vi "IT6900 Run List.vi"() -> ()   [LabVIEW 2013]
uses:
  IT6900.lvlib
panel:
  in  "List Step Count":i32=2 min=1
  in  "Loop count":i32=1 min=0
  in  "List Timer":i32=3 min=0
  in  "Trigger Current Limit (0.0 A)":dbl format="%.2g"
  in  "Trigger Voltage Limit (0.0 V)":dbl format="%.2g"
  in  "List Save Region":i8 min=0 max=9
  in  "Serial Configuration":T1={"Baud Rate"=9600, "Parity"=0, "Data Bits"=8, "Stop Bits"=10, "Flow Control"=0} {"Flow Control" items=["None", "XON/XOFF", "RTS/CTS", "XON/XOFF & RTS/CTS", "DTR/DSR", "XON/XOFF & DTR/DSR"]; "Stop Bits" items=["1.0"=10, "1.5"=15, "2.0"=20]; "Data Bits" items=["7"=7, "8"=8]; "Parity" items=["None", "Odd", "Even", "Mark", "Space"]; "Baud Rate" items=["300"=300, "600"=600, "1200"=1200, "2400"=2400, "4800"=4800, "9600"=9600, "19200"=19200]}
  in  "VISA resource name":refnum<visa-resource-name>
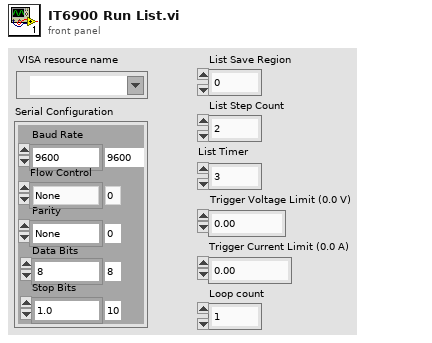
[diagram p1: front panel]
types:
  T1 = cluster{"Baud Rate":u32, "Parity":u16, "Data Bits":u16, "Stop Bits":u16, "Flow Control":u16}
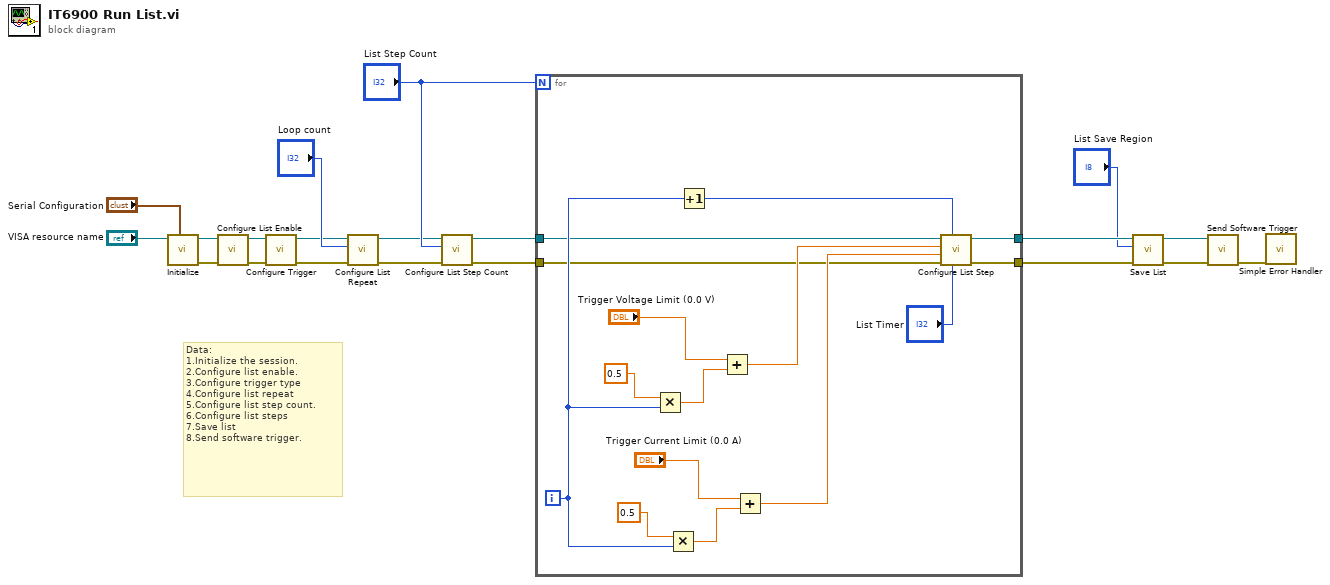
[diagram p0: block diagram]
diagram:
  # "Data:\n1.Initialize the session.\n2.Configure list enable.\n3.Configure trigger type\n4.Configure list repeat\n5.Configure list step count.\n6.Configure list steps\n7.Save list\n8.Send software trigger."
  n1 = call "Initialize.vi"("Serial Configuration"="Serial Configuration", "VISA resource name"="VISA resource name") -> ("error out"=w9:errorcluster, "VISA resource name out"=w10:refnum<visa-resource-name>)  [unwired: 8 in]
  n2 = call "Configure List Enable.vi"("error in (no error)"=w9, "VISA resource name"=w10) -> ("error out"=w8:errorcluster, "VISA resource name out"=w7:refnum<visa-resource-name>)  [unwired: 8 in]
  n3 = call "Configure Trigger.vi"("error in (no error)"=w8, "VISA resource name"=w7) -> ("error out"=w5:errorcluster, "VISA resource name out"=w6:refnum<visa-resource-name>)  [unwired: 8 in]
  n4 = call "Configure List Repeat.vi"("error in (no error)"=w5, "Loop count (1)"="Loop count", "VISA resource name"=w6) -> ("error out"=w3:errorcluster, "VISA resource name out"=w4:refnum<visa-resource-name>)  [unwired: 7 in]
  n5 = call "Configure List Step Count.vi"("error in (no error)"=w3, "List Total"="List Step Count", "VISA resource name"=w4) -> ("error out"=w12:errorcluster, "VISA resource name out"=w13:refnum<visa-resource-name>)  [unwired: 7 in]
  n6 = for {
    N: "List Step Count" -> [_]
    tunnel: w13 -> [w25]
    tunnel: w12 -> [w24]
    tunnel: [w23] -> w18
    tunnel: [w22] -> w17
    i -> [w27]
    n7 = Multiply(x=0.5, y=w27) -> (x*y=w34:dbl)
    n8 = Multiply(x=0.5, y=w27) -> (x*y=w30:dbl)
    n9 = Increment(x=w27) -> (x+1=w26:i32)
    n10 = Add(x="Trigger Voltage Limit (0.0 V)", y=w34) -> (x+y=w32:dbl)
    n11 = Add(x="Trigger Current Limit (0.0 A)", y=w30) -> (x+y=w28:dbl)
    n12 = call "Configure List Step.vi"("List Timer"="List Timer", "List Index"=w26, "error in (no error)"=w24, "Trigger Current Limit (0.0 A)"=w28, "Trigger Voltage Limit (0.0 V)"=w32, "VISA resource name"=w25) -> ("error out"=w22:errorcluster, "VISA resource name out"=w23:refnum<visa-resource-name>)  [unwired: 4 in]
  }
  n13 = call "Save List.vi"("error in (no error)"=w17, "Save Region (0)"="List Save Region", "VISA resource name"=w18) -> ("error out"=w1:errorcluster, "VISA resource name out"=w2:refnum<visa-resource-name>)  [unwired: 7 in]
  n14 = call "Send Software Trigger.vi"("error in (no error)"=w1, "VISA resource name"=w2) -> ("error out"=w14:errorcluster)  [unwired: 8 in, 1 out]
  n15 = call <vilib>:"Simple Error Handler.vi"("error in (no error)"=w14) -> ()  [unwired: 4 in, 5 out]
